vi "Pump_destage.vi"(0 "Start":bool, 1 "N_pump_on":u32, 2 "N_pump_on_ref":u32, 3 "Num_pump_on_ref":u32, 4 "N_pump":u32, 7 "T_pump_on_time":u32, 9 "N_pump_on_ref_alr":bool) -> (14 "N curr":u32, 15 "-1":bool, 16 "ok":bool, 17 "not ok":bool, 18 "t":u32)   [LabVIEW 2019]
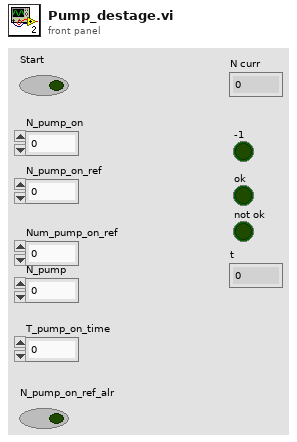
[diagram p1: front panel]
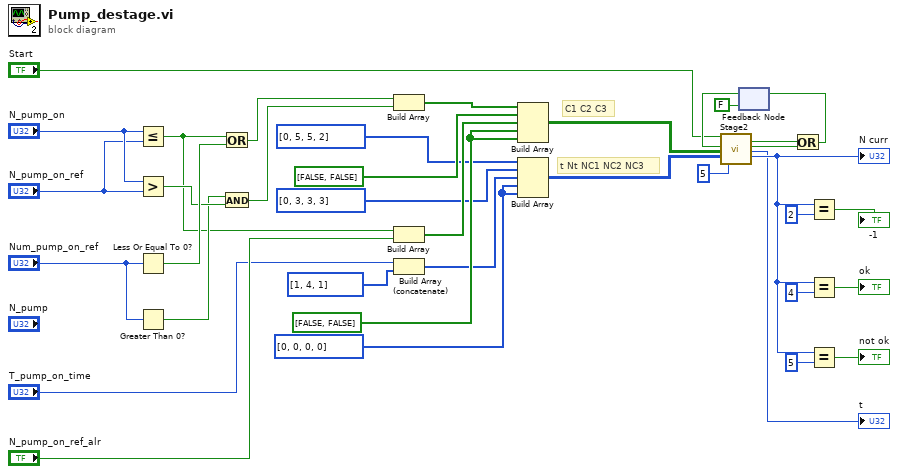
[diagram p0: block diagram]
diagram:
  w12 = u32[] [0, 0, 0, 0] ("Stage table")
  w11 = bool[] [FALSE, FALSE]
  # "C1 C2 C3"
  # "t Nt NC1 NC2 NC3"
  n1 = Less Or Equal?(x="N_pump_on", y="N_pump_on_ref") -> (x <= y?=w25:bool)
  n2 = Greater?(x="N_pump_on", y="N_pump_on_ref") -> (0:w32:bool)
  n3 = Less Or Equal To 0?(x="Num_pump_on_ref") -> (x <= 0?=w33:bool)
  n4 = Greater Than 0?(x="Num_pump_on_ref") -> (x > 0?=w31:bool)
  n5 = Or(x=w25, y=w33) -> (x .or. y?=w3:bool)
  n6 = And(x=w31, y=w32) -> (x .and. y?=w28:bool)
  n7 = Build Array(w3, w28) -> (w6:bool[])
  n8 = Build Array(w25, "N_pump_on_ref_alr") -> (w9:bool[])
  n9 = Build Array (concatenate)("T_pump_on_time", u32[] [1, 4, 1] ("Stage table")) -> (w10:u32[])
  n10 = Build Array(w6, bool[] [FALSE, FALSE], w9, w11, w11) -> (w27:bool[][])
  n11 = Build Array(u32[] [0, 5, 5, 2] ("Stage table"), u32[] [0, 3, 3, 3] ("Stage table"), w10, w12, w12) -> (w21:u32[][])
  n12 = feedback #1(FALSE) -> (w34:bool)
  n13 = call "Stage2.vi"("Start"="Start", "Reset"=w34, "C"=w27, "Stage table"=w21, "End step"=u32 5) -> ("Stop"=w37:bool, "End"=w36:bool, "t"=→"t":u32, "N curr"=w20:u32)  [unwired: 9 in, 2 out]
  "N curr" <- w20
  n14 = Or(x=w37, y=w36) -> (x .or. y?=w35:bool)
  n15 = feedback-in #1(w35) -> ()
  n16 = Equal?(x=w20, y=u32 2) -> (x = y?=→"-1":bool)
  n17 = Equal?(x=w20, y=u32 4) -> (x = y?=→"ok":bool)
  n18 = Equal?(x=w20, y=u32 5) -> (x = y?=→"not ok":bool)
